vi "Index of Mods in Sp ID Array.vi"(8 "error in (no error)":errorcluster, 10 "Sp_Id_Arr":string[](array[string]), 11 "Ex_Mod_IDs":string[](array[string])) -> (0 "error out":errorcluster, 2 "Idx of Mod in Sp IDs":i32[](array[numeric]))   [LabVIEW 2014]
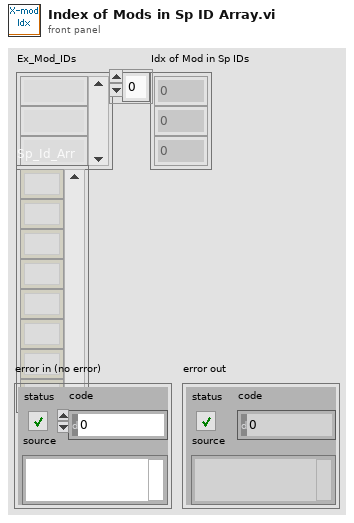
[diagram p1: front panel]
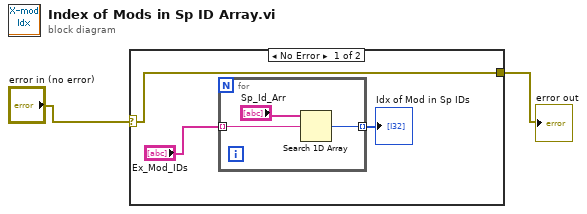
[diagram p0: block diagram]
diagram:
  n1 = case shown="No Error" "error in (no error)" {
    selector: "error in (no error)" -> [w3 w9]
    tunnel: [w3 w9] -> w1
    frame No Error {
      n2 = for {
        tunnel: "Ex_Mod_IDs" -> [w7] mode=indexing
        tunnel: [w6] -> w4 mode=indexing
        n3 = Search 1D Array(1D array="Sp_Id_Arr", element=w7) -> (index of element=w6:i32)  [unwired: 1 in]
      }
      "Idx of Mod in Sp IDs" <- w4
    }
    frame Error {
    }
  }
  "error out" <- w1
